vi "Voltech PM1000+ Standby Measurement.vi"() -> ()   [LabVIEW 2015]
doc: "The purpose of this vi is to show the basic measurements that PM1000+ can make. The results are returned using the FRD command. This returns the results that are shown on the screen, in the order in which they appear on the screen. As results are selected using comms, the results are added to the bottom of the list, with the exception of harmonics, which always appear at the end of the list."
uses:
  <vilib>/Utility/error.llb/DialogType.ctl
  <instrlib>/Voltech PM1000+/Public/Configure/Configure Measurements (Standby).vi
  <instrlib>/Voltech PM1000+/Voltech PM1000+.lvlib
panel:
  in  "Reset (True)":bool=TRUE
  in  "ID Query (True)":bool=TRUE
  in  "Serial Configuration":T1={"Baud Rate"=19200, "Parity"=0, "Data Bits"=8, "Stop Bits"=10, "Flow Control"=2} {"Flow Control" items=["None"=0, "RTS/CTS"=2]; "Stop Bits" items=["1.0"=10]; "Data Bits" items=["8"=8]; "Parity" items=["None"]; "Baud Rate" items=["9600"=9600, "19200"=19200, "38400"=38400]}
  in  "Measurements":T2={"Voltage Harmonics"={"Range (7)"=7.0, "Sequence (Odd & Even)"=0}, "Averaging Period (10s)"=5, "Measurements - Standby"=[0, 1, 2, 5, 6, 7, 8]} {"Averaging Period (10s)" min=1 max=300 step=1; "Voltage Harmonics"."Sequence (Odd & Even)" items=["Odd & Even", "Odd Only"]; "Voltage Harmonics"."Range (7)" min=1.0 max=50.0 step=1.0}
  out "Number of Measurements Taken":u32
  in  "Select Mode (Normal)":u16(ring)=3 items=["Normal", "Ballast", "Inrush", "Standby Power", "Integrator"]
  in  "Enable Autozero  (True)":bool=TRUE caption="Autozero  (Enable)"
  in  "Enable Blanking (True)":bool=TRUE
  in  "Shunt (Internal)":u16(ring) items=["Internal", "External"]
  in  "Freq Source (Voltage)":u16(ring) items=["Voltage", "Current"]
  in  "Fixed/Auto Ranging":T3 {"Volts Ranging (Auto)" items=["Auto", "10Vpk", "46Vpk", "215Vpk", "900Vpk"]; "Amps Ranging (Auto)" items=["Auto", "0.1Apk", "0.4Apk", "1.6Apk", "6.25Apk", "25Apk", "100Apk"]}
  in  "Scaling":T4={"Voltage Sacling (1.0000)"=1.0, "Current Sacling (1.0000)"=1.0} {"Current Sacling (1.0000)" min=1e-06 max=1000000.0 step=1.0 format="%.6f"; "Voltage Sacling (1.0000)" min=1e-06 max=1000000.0 step=1.0 format="%.6f"}
  in  "VISA resource name":refnum<visa-resource-name>
  in  "stop":bool
  out "Parameter":string[](array[string])
  out "Value":dbl[](array[numeric])
  # "(c) 2008-2009 Voltech Instruments.  ALL RIGHTS RESERVED."
  # "Configuration Side"
  # "1. Leave it as default or set up the PM1000+ instruments on the left  \n    \"Configuration Side\".\n2. Press Ctrl+R to run the test.\n3. Press the lower right side \"STOP\" button to stop the test."
  # "Sec (1~100)"
  # "1~50"
  # "Results Side"
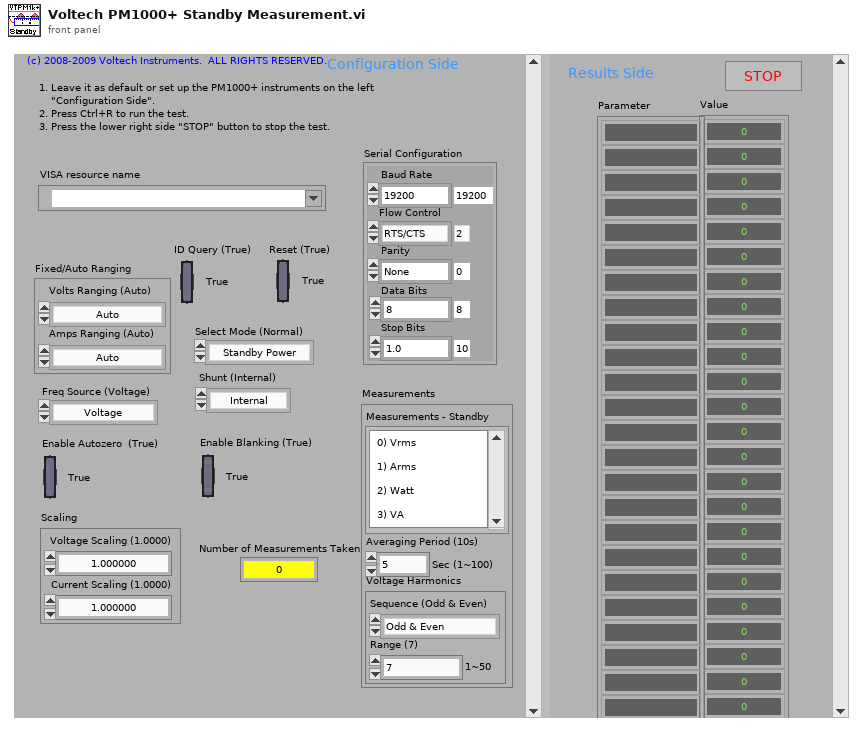
[diagram p1: front panel]
types:
  T1 = cluster{"Baud Rate":u32, "Parity":u16, "Data Bits":u16, "Stop Bits":u16, "Flow Control":u16}
  T2 = cluster{"Voltage Harmonics":cluster{"Range (7)":dbl, "Sequence (Odd & Even)":u16}, "Averaging Period (10s)":i32, "Measurements - Standby":i32[]}
  T3 = cluster{"Amps Ranging (Auto)":u16, "Volts Ranging (Auto)":u16}
  T4 = cluster{"Voltage Sacling (1.0000)":dbl, "Current Sacling (1.0000)":dbl}
  T5 = typedef "DialogType.ctl" = u16
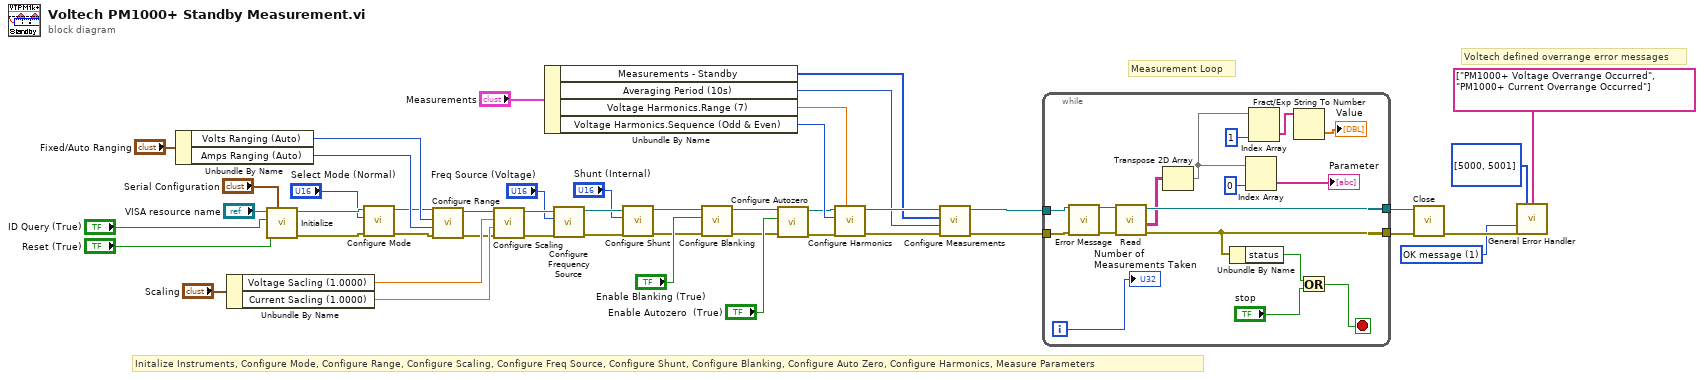
[diagram p0: block diagram]
diagram:
  w14 = T5 1 items=["no dialog", "OK message", "continue or stop message", "OK message + warnings", "continue/stop + warnings"] ("type of dialog (OK msg:1)")
  # "Initalize Instruments, Configure Mode, Configure Range, Configure Scaling, Configure Freq Source, Configure Shunt, Configure Blanking, Configure Auto Zero, Configure Harmonics, Measure Parameters"
  # "Measurement Loop"
  # "Voltech defined overrange error messages"
  n1 = Unbundle By Name("Fixed/Auto Ranging") -> ("Volts Ranging (Auto)"=w37:u16, "Amps Ranging (Auto)"=w36:u16)
  n2 = Unbundle By Name("Scaling") -> ("Voltage Sacling (1.0000)"=w40:dbl, "Current Sacling (1.0000)"=w39:dbl)
  n3 = call <instrlib>:"Initialize.vi"("Serial Configuration"="Serial Configuration", "Reset (True)"="Reset (True)", "ID Query (True)"="ID Query (True)", "VISA resource name"="VISA resource name") -> ("error out"=w6:errorcluster, "VISA resource name out"=w7:refnum<visa-resource-name>)  [unwired: 6 in]
  n4 = call <instrlib>:"Configure Mode.vi"("error in (no error)"=w6, "Select Mode (Normal)"="Select Mode (Normal)", "VISA resource name"=w7) -> ("error out"=w4:errorcluster, "VISA resource name out"=w5:refnum<visa-resource-name>)  [unwired: 7 in]
  n5 = call <instrlib>:"Configure Range.vi"("error in (no error)"=w4, "Current Range (Auto)"=w36, "Voltage Range (Auto)"=w37, "VISA resource name"=w5) -> ("error out"=w8:errorcluster, "VISA resource name out"=w9:refnum<visa-resource-name>)  [unwired: 6 in]
  n6 = call <instrlib>:"Configure Scaling.vi"("error in (no error)"=w8, "Current Sacling (1.0000)"=w39, "Voltage Sacling (1.0000)"=w40, "VISA resource name"=w9) -> ("error out"=w42:errorcluster, "VISA resource name out"=w43:refnum<visa-resource-name>)  [unwired: 6 in]
  n7 = Unbundle By Name("Measurements") -> ("Measurements - Standby"=w20:i32[], "Averaging Period (10s)"=w19:i32, "Voltage Harmonics.Range (7)"=w17:dbl, "Voltage Harmonics.Sequence (Odd & Even)"=w18:u16)
  n8 = call <instrlib>:"Configure Frequency Source.vi"("error in (no error)"=w42, "Frequency Source (Voltage)"="Freq Source (Voltage)", "VISA resource name"=w43) -> ("error out"=w45:errorcluster, "VISA resource name out"=w44:refnum<visa-resource-name>)  [unwired: 7 in]
  n9 = call <instrlib>:"Configure Shunt.vi"("error in (no error)"=w45, "Shunt (Internal)"="Shunt (Internal)", "VISA resource name"=w44) -> ("error out"=w25:errorcluster, "VISA resource name out"=w24:refnum<visa-resource-name>)  [unwired: 7 in]
  n10 = call <instrlib>:"Configure Blanking.vi"("error in (no error)"=w25, "Enable Blanking (True)"="Enable Blanking (True)", "VISA resource name"=w24) -> ("error out"=w22:errorcluster, "VISA resource name out"=w23:refnum<visa-resource-name>)  [unwired: 7 in]
  n11 = call <instrlib>:"Configure Autozero.vi"("error in (no error)"=w22, "Enable Autozero (True)"="Enable Autozero  (True)", "VISA resource name"=w23) -> ("error out"=w10:errorcluster, "VISA resource name out"=w11:refnum<visa-resource-name>)  [unwired: 7 in]
  n12 = call <instrlib>:"Configure Harmonics.vi"("Voltage Harmonic Range (7)"=w17, "error in (no error)"=w10, "Voltage Harmonic Sequence (Odd & Even)"=w18, "VISA resource name"=w11) -> ("error out"=w33:errorcluster, "VISA resource name out"=w34:refnum<visa-resource-name>)  [unwired: 6 in]
  n13 = call-poly <instrlib>:"Configure Measurements.vi"("error in (no error)"=w33, "Averaging Period (10sec)"=w19, "Standby Measurements"=w20, "VISA resource name"=w34) -> ("error out"=w29:errorcluster, "VISA resource name out"=w30:refnum<visa-resource-name>)  [unwired: 6 in]
  n14 = while {
    tunnel: w30 -> [w48]
    tunnel: w29 -> [w47]
    tunnel: [w63] -> w28
    tunnel: [w54] -> w27
    i -> [w62]
    stop <- w51 stop-if-true
    n15 = call <instrlib>:"Error Message.vi"("VISA resource name"=w48, "error in (no error)"=w47) -> ("VISA resource name out"=w50:refnum<visa-resource-name>, "error out"=w49:errorcluster)  [unwired: 12 in]
    n16 = call <instrlib>:"Read.vi"("error in (no error)"=w49, "VISA resource name"=w50) -> ("error out"=w54:errorcluster, "Measurement Results"=w61:string[][], "VISA resource name out"=w63:refnum<visa-resource-name>)  [unwired: 7 in]
    n17 = Transpose 2D Array(2D array=w61) -> (transposed array=w60:string[][])
    n18 = Unbundle By Name(w54) -> ("status"=w53:bool)
    n19 = Index Array(array=w60, index (col)=0) -> (element=→"Parameter":string[])  [unwired: 1 in]
    n20 = Index Array(array=w60, index (col)=1) -> (element=w59:string[])  [unwired: 1 in]
    n21 = Fract/Exp String To Number(string=w59) -> (number=→"Value":dbl[])  [unwired: 3 in, 1 out]
    n22 = Or(x=w53, y="stop") -> (x .or. y?=w51:bool)
    "Number of Measurements Taken" <- w62
  }
  n23 = call <instrlib>:"Close.vi"("error in (no error)"=w27, "VISA resource name"=w28) -> ("error out"=w15:errorcluster)  [unwired: 9 in]
  n24 = call <vilib>:"General Error Handler.vi"("[user-defined codes]"=i32[] [5000, 5001], "[user-defined descriptions]"=string[] ["PM1000+ Voltage Overrange Occurred", "PM1000+ Current Overrange Occurred"], "type of dialog (OK msg:1)"=w14, "error in (no error)"=w15) -> ()  [unwired: 7 in, 5 out]
